vi "main.vi"() -> ()   [LabVIEW 2020]
uses:
  Typedefs/Queue_Operations.ctl
  Typedefs/Data Cluster.ctl
  Typedefs/Timer.ctl
  <vilib>/Utility/config.llb/Read Key (Double).vi
  <vilib>/Utility/config.llb/Write Key (Double).vi
  <vilib>/Utility/config.llb/NI_LVConfig.lvlib
panel:
  out "Milk Level":dbl(slide)=70.0 scale=0.0..100.0
  out "Bean Level":dbl(slide)=70.0 scale=0.0..100.0
  out "Water Level":dbl(slide)=70.0 scale=0.0..100.0
  in  "Power":bool
  out "Total Cups":dbl
  out "Elapsed Time":i32
  out "Dispensing":bool
  out "Brewing":bool
  out "Grinding":bool
  out "Heating":bool
  out "Purging":bool
  out "Dispenser":dbl(slide) scale=0.0..60.0
  out "Chamber":dbl(slide) scale=0.0..60.0
  out "Low Milk":bool
  out "Low Bean":bool
  out "Low Water":bool
  in  "Knob":i32(knob)=2 scale=0.0..2.0
  in  "1 Carafe":bool
  in  "1 Cup":bool
  out "Error out":errorcluster
  in  "Error in":errorcluster
  # "Coffee"
  # "Hot Water"
  # "Lattee"
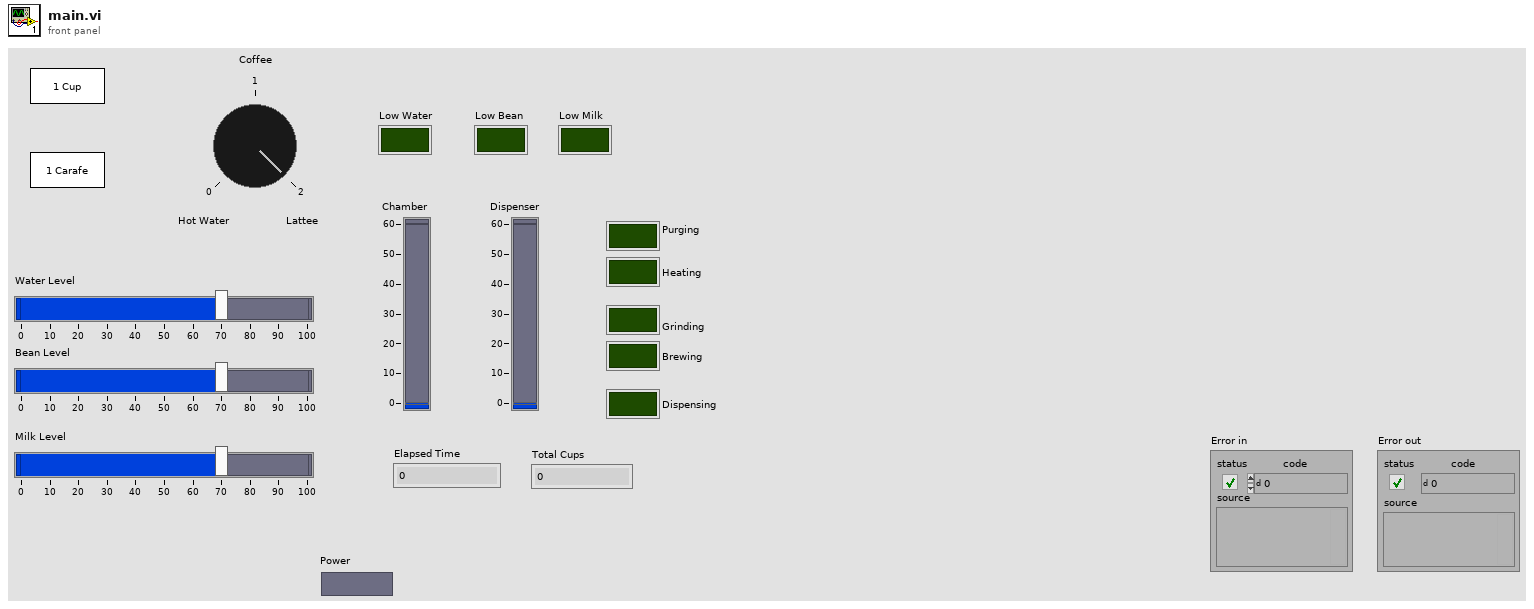
[diagram p1: front panel]
types:
  T1 = typedef "Data Cluster.ctl" = cluster{"Timer":T2, "Power":bool, "Total Cups":dbl, "Coffee Path":path, "Shut Down":dbl, "Water Level":dbl, "Bean Level":dbl, "Milk Level":dbl, "Knob":i32, "Beverage Type":string, "1 Cup":bool, "1 Carafe":bool, "Chamber":dbl, "Dispenser":dbl, "Set Time":dbl[], "Sequence":cluster{"Ingri":string, "Time":dbl}[], "index":i32, "Purging":bool, "Heating":bool, "Grinding":bool, "Brewing":bool, "Dispensing":bool, "Low Water":bool, "Low Bean":bool, "Low Milk":bool}
  T2 = typedef "Timer.ctl" = cluster{"Previous Time":dbl, "Elapsed Time":dbl, "Start":bool, "Pause?":bool}
  T3 = typedef "Queue_Operations.ctl" = enum16{"Obtain Queue", "Enqueue", "Enqueue N Element", "Enqueue at First", "Dequeue", "Release Queue", "Queue Status", "Flush Queue"}
  T4 = typedef "NI_LVConfig.lvlib/Config Data RefNum.ctl" = refnum<k1>
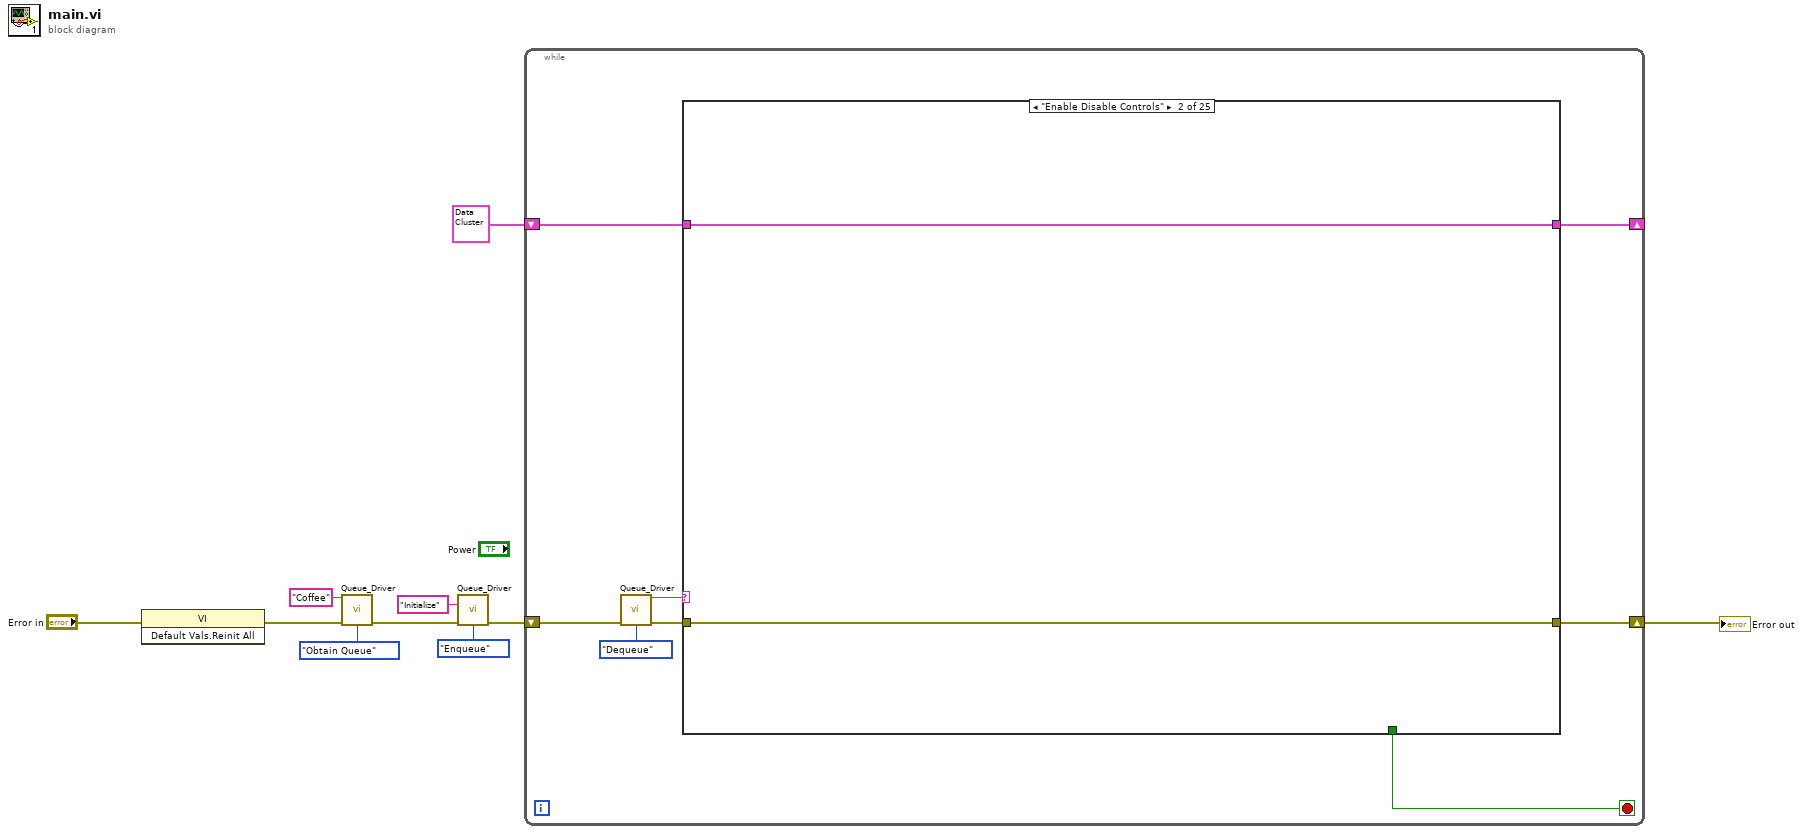
[diagram p0: block diagram]
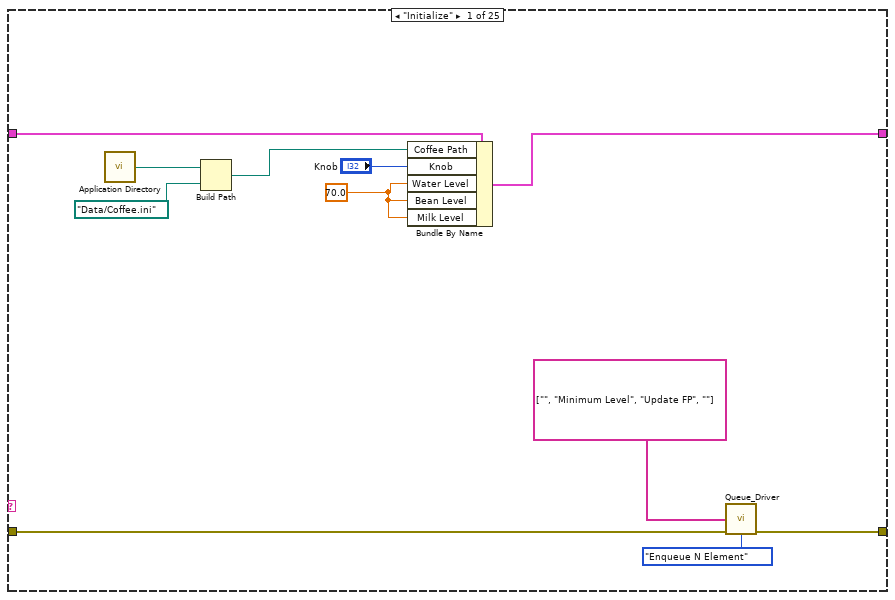
[diagram p2: hidden frame]
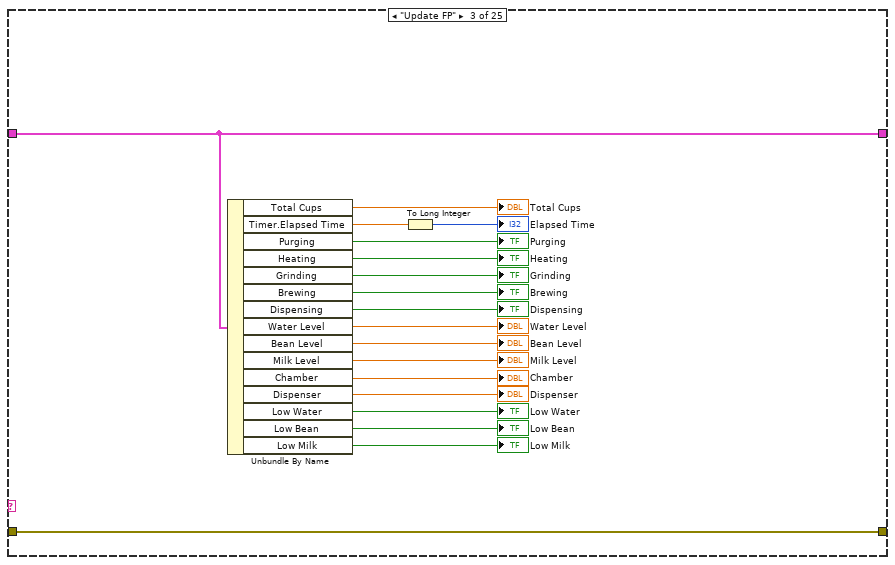
[diagram p3: hidden frame]
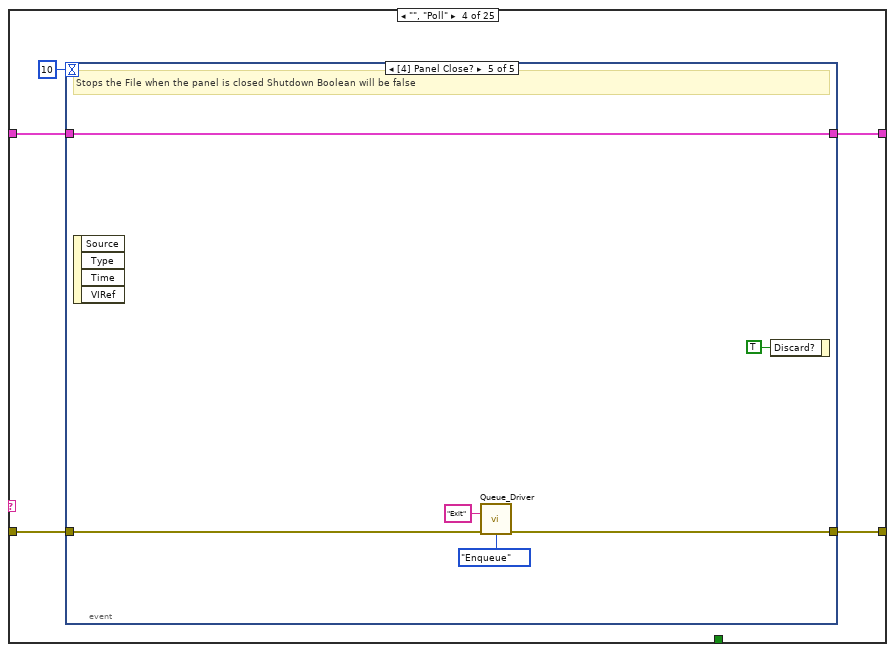
[diagram p4: hidden frame]
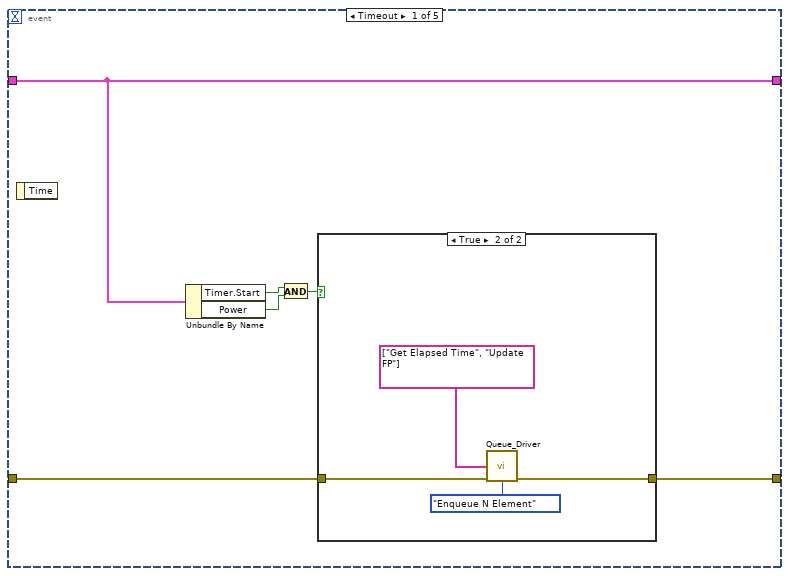
[diagram p5: hidden frame]
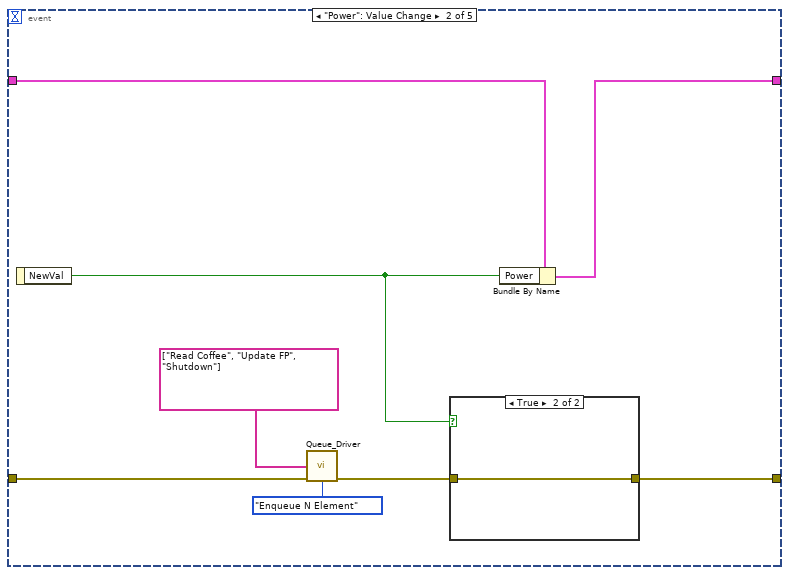
[diagram p7: hidden frame]
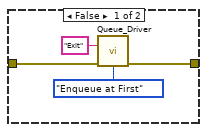
[diagram p8: hidden frame]
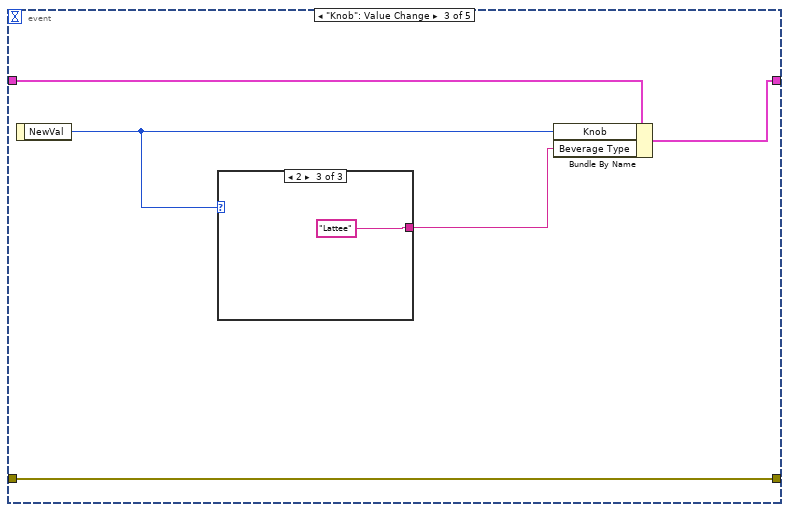
[diagram p9: hidden frame]
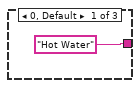
[diagram p10: hidden frame]
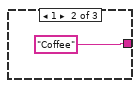
[diagram p11: hidden frame]
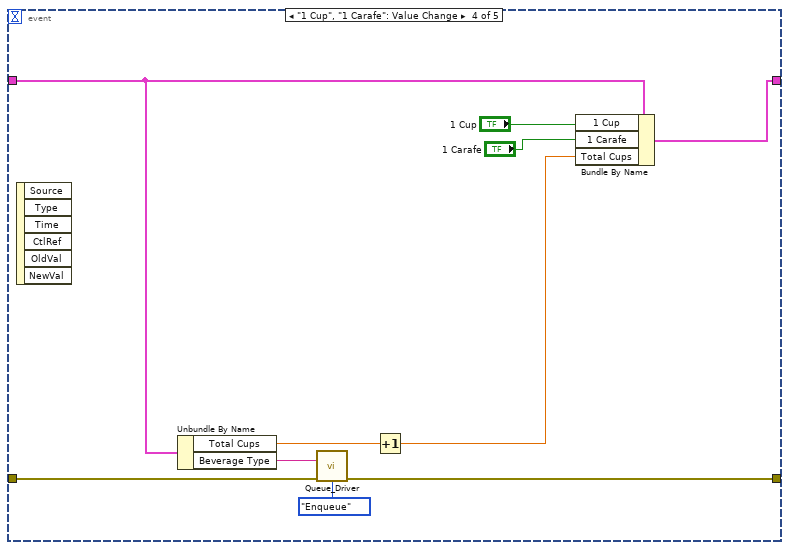
[diagram p12: hidden frame]
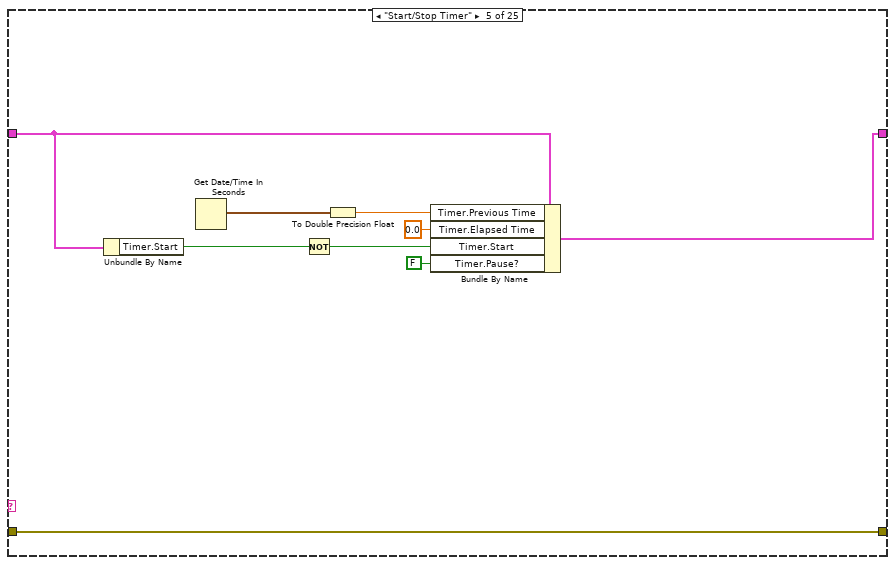
[diagram p13: hidden frame]
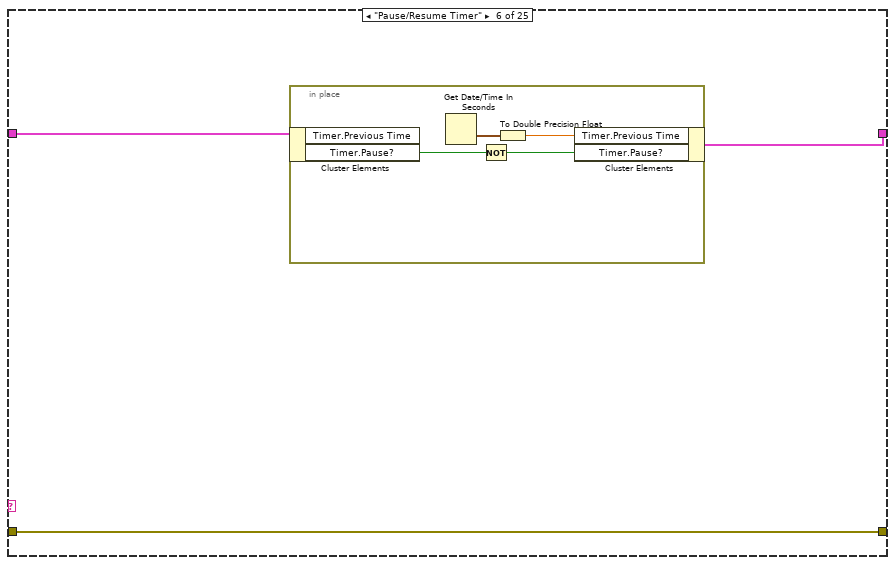
[diagram p14: hidden frame]
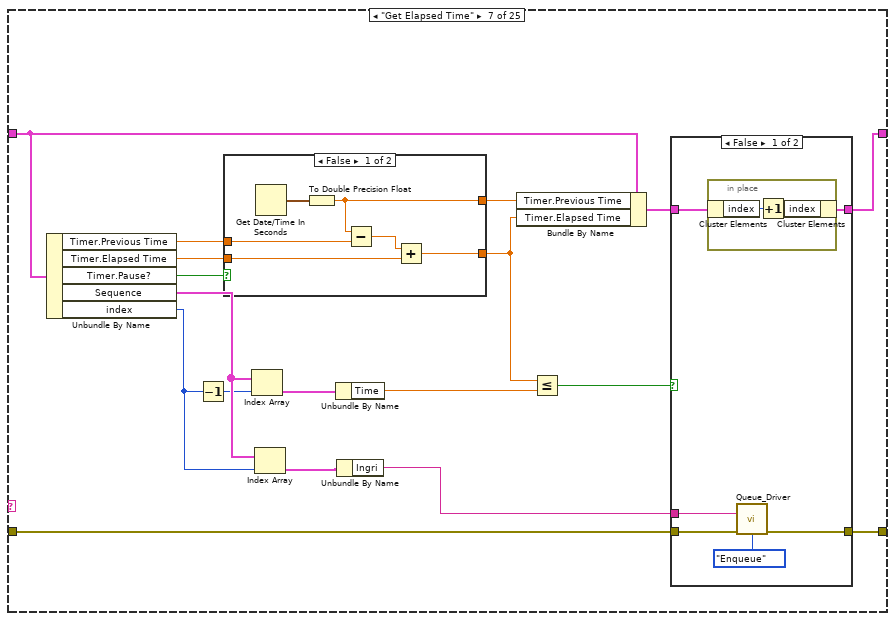
[diagram p15: hidden frame]
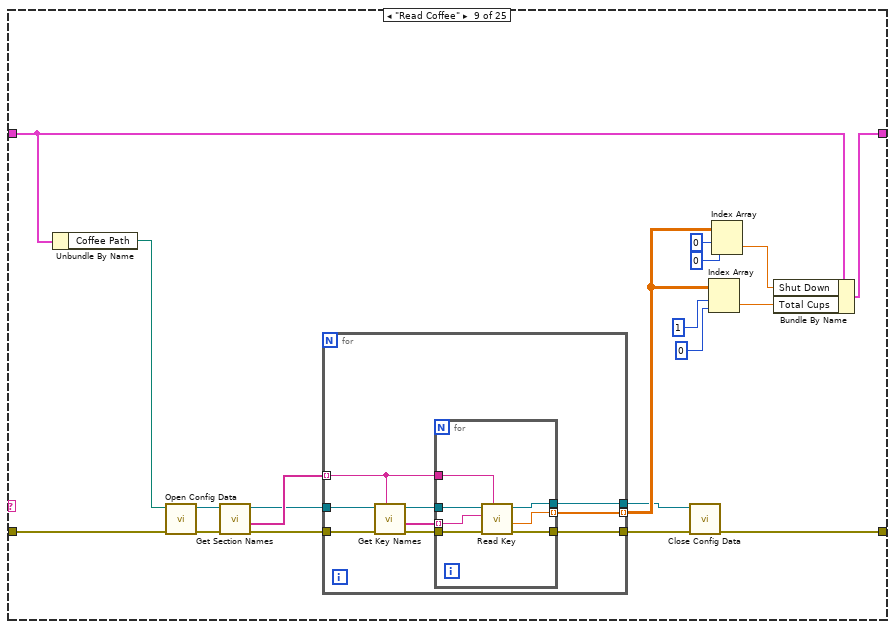
[diagram p19: hidden frame]
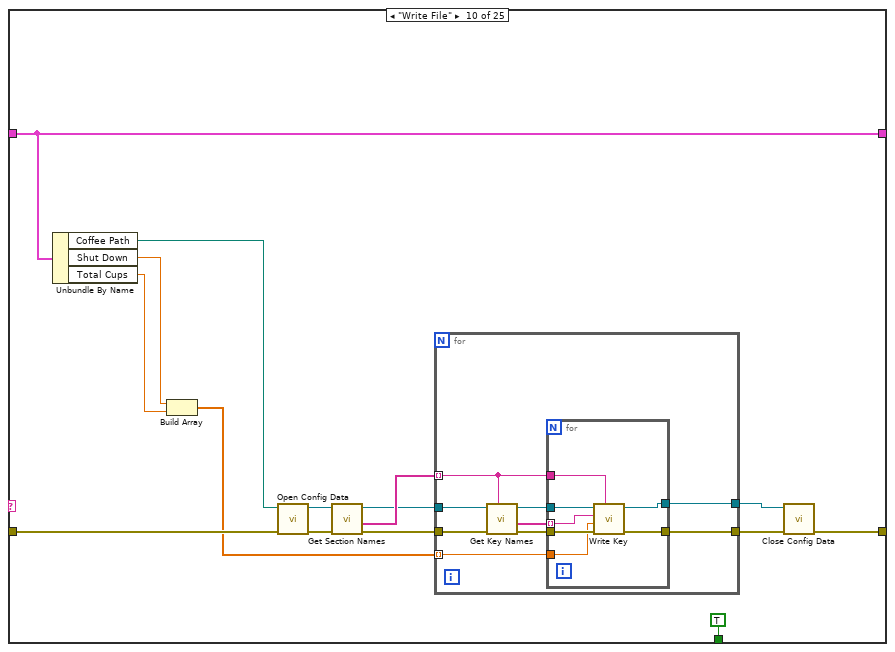
[diagram p20: hidden frame]
diagram:
  n1 = invoke class="VI" method="Default Vals.Reinit All"(error in="Error in") -> (error out=w1:errorcluster)  [unwired: 2 in, 2 out]
  n2 = call "Queue_Driver.vi"("Queue Name"="Coffee", "error in (no error)"=w1, "Queue Operation"=Queue_Operations."Obtain Queue") -> ("error out"=w6:errorcluster)  [unwired: 11 in, 1 out]
  n3 = call "Queue_Driver.vi"("Enqueue State"="Initialize", "error in (no error)"=w6, "Queue Operation"=Queue_Operations."Enqueue") -> ("error out"=w5:errorcluster)  [unwired: 11 in, 1 out]
  n4 = while {
    shift-right: [w18] -> w10
    shift-left: w5 -> [w17]
    shift-right: [w13] -> _
    shift-left: T1 {"Timer"={"Previous Time"=0.0, "Elapsed Time"=0.0, "Start"=FALSE, "Pause?"=FALSE}, "Power"=FALSE, "Total Cups"=0.0, "Coffee Path"=path "", "Shut Down"=0.0, "Water Level"=0.0, "Bean Level"=0.0, "Milk Level"=0.0, "Knob"=0, "Beverage Type"="", "1 Cup"=FALSE, "1 Carafe"=FALSE, "Chamber"=0.0, "Dispenser"=0.0, "Set Time"=[], "Sequence"=[{"Ingri"="Beverage Type", "Time"=0.0}], "index"=1, "Purging"=FALSE, "Heating"=FALSE, "Grinding"=FALSE, "Brewing"=FALSE, "Dispensing"=FALSE, "Low Water"=FALSE, "Low Bean"=FALSE, "Low Milk"=FALSE} ("Data Cluster") -> [w12]
    stop <- w11 stop-if-true
    n5 = call "Queue_Driver.vi"("error in (no error)"=w17, "Queue Operation"=Queue_Operations."Dequeue") -> ("Dequeued State"=w14:string, "error out"=w16:errorcluster)  [unwired: 12 in]
    n6 = case shown="\"Enable Disable Controls\"" w14 {
      tunnel: w16 -> [w23 w30 w49 w54 w103 w112 w130 w155 w172 w205 w229 w250 w255 w263 w272 w281 w306 w327 w358 w365 w374 w380 w390 w396 w398]
      tunnel: [w24 w30 w49 w53 w103 w112 w131 w155 w158 w194 w223 w250 w254 w262 w271 w281 w306 w327 w358 w365 w374 w379 w389 w396 w398] -> w18
      tunnel: [w28 w31 w48 w51 w111 w113 w120 w156 w175 w199 w232 w244 w257 w265 w274 w280 w308 w330 w359 w363 w373 w384 w393 w397 w399] -> w13
      tunnel: w12 -> [w29 w31 w48 w52 w106 w114 w133 w156 w174 w199 w234 w245 w258 w266 w268 w276 w303 w324 w354 w364 w367 w382 w395 w397 w399]
      tunnel: [_ _ _ _ _ _ _ _ _ TRUE _ _ _ _ _ _ _ _ _ _ _ _ FALSE _ _] -> w11
      frame "Initialize" {
        w19 = 70.0 ("Water Level")
        n7 = call <vilib>:"Application Directory.vi"() -> ("Application Directory"=w27:path)
        n8 = Build Path(base path=w27, name or relative path=path "Data/Coffee.ini") -> (appended path=w25:path)
        n9 = Bundle By Name(cluster=w29, "Coffee Path"=w25, "Knob"="Knob", "Water Level"=w19, "Bean Level"=w19, "Milk Level"=w19) -> (w28:T1)
        n10 = call "Queue_Driver.vi"("Array of States"=string[] ["", "Minimum Level", "Update FP", ""], "error in (no error)"=w23, "Queue Operation"=Queue_Operations."Enqueue N Element") -> ("error out"=w24:errorcluster)  [unwired: 11 in, 1 out]
      }
      frame "Enable Disable Controls" {
      }
      frame "Update FP" {
        n11 = Unbundle By Name(w48) -> ("Total Cups"=→"Total Cups":dbl, "Timer.Elapsed Time"=w47:dbl, "Purging"=→"Purging":bool, "Heating"=→"Heating":bool, "Grinding"=→"Grinding":bool, "Brewing"=→"Brewing":bool, "Dispensing"=→"Dispensing":bool, "Water Level"=→"Water Level":dbl, "Bean Level"=→"Bean Level":dbl, "Milk Level"=→"Milk Level":dbl, "Chamber"=→"Chamber":dbl, "Dispenser"=→"Dispenser":dbl, "Low Water"=→"Low Water":bool, "Low Bean"=→"Low Bean":bool, "Low Milk"=→"Low Milk":bool)
        n12 = To Long Integer(number=w47) -> (32bit integer=→"Elapsed Time":i32)
      }
      frame "", "Poll" {
        n13 = event shown="[4] Panel Close?" {
          selector: _ -> [_ _ _ _ _]
          dyn-events: _ -> [_ _ _ _ _]
          timeout: 10 -> [_ _ _ _ _]
          tunnel: w54 -> [w60 w71 w81 w96 w100]
          tunnel: [w59 w67 w81 w95 w99] -> w53
          tunnel: w52 -> [w58 w73 w83 w92 w102]
          tunnel: [w58 w72 w82 w91 w102] -> w51
          event Timeout {
            n14 = event-data() -> ()  [unwired: 1 in, 1 out]
            n15 = Unbundle By Name(w58) -> ("Timer.Start"=w56:bool, "Power"=w55:bool)
            n16 = And(x=w56, y=w55) -> (x .and. y?=w57:bool)
            n17 = case shown="True" w57 {
              tunnel: w60 -> [w61 w65]
              tunnel: [w61 w64] -> w59
              frame False {
              }
              frame True {
                n18 = call "Queue_Driver.vi"("Array of States"=string[] ["Get Elapsed Time", "Update FP"], "error in (no error)"=w65, "Queue Operation"=Queue_Operations."Enqueue N Element") -> ("error out"=w64:errorcluster)  [unwired: 11 in, 1 out]
              }
            }
          }
          event "Power": Value Change {
            n19 = event-data() -> ("NewVal"=w66:bool)  [unwired: 1 in]
            n20 = call "Queue_Driver.vi"("Array of States"=string[] ["Read Coffee", "Update FP", "Shutdown"], "error in (no error)"=w71, "Queue Operation"=Queue_Operations."Enqueue N Element") -> ("error out"=w68:errorcluster)  [unwired: 11 in, 1 out]
            n21 = case shown="True" w66 {
              tunnel: w68 -> [w77 w78]
              tunnel: [w76 w78] -> w67
              frame False {
                n22 = call "Queue_Driver.vi"("Enqueue State"="Exit", "error in (no error)"=w77, "Queue Operation"=Queue_Operations."Enqueue at First") -> ("error out"=w76:errorcluster)  [unwired: 11 in, 1 out]
              }
              frame True {
              }
            }
            n23 = Bundle By Name(cluster=w73, "Power"=w66) -> (w72:T1)
          }
          event "Knob": Value Change {
            n24 = event-data() -> ("NewVal"=w80:i32)  [unwired: 1 in]
            n25 = case shown="2" w80 {
              tunnel: ["Hot Water" "Coffee" "Lattee"] -> w79
              frame 0, Default {
              }
              frame 1 {
              }
              frame 2 {
              }
            }
            n26 = Bundle By Name(cluster=w83, "Knob"=w80, "Beverage Type"=w79) -> (w82:T1)
          }
          event "1 Cup", "1 Carafe": Value Change {
            n27 = event-data() -> ()  [unwired: 1 in, 6 out]
            n28 = Unbundle By Name(w92) -> ("Total Cups"=w88:dbl, "Beverage Type"=w93:string)
            n29 = call "Queue_Driver.vi"("Enqueue State"=w93, "error in (no error)"=w96, "Queue Operation"=Queue_Operations."Enqueue") -> ("error out"=w95:errorcluster)  [unwired: 11 in, 1 out]
            n30 = Increment(x=w88) -> (x+1=w87:dbl)
            n31 = Bundle By Name(cluster=w92, "1 Cup"="1 Cup", "1 Carafe"="1 Carafe", "Total Cups"=w87) -> (w91:T1)
          }
          event Panel Close? {
            # "Stops the File when the panel is closed Shutdown Boolean will be false"
            n32 = event-data() -> ()  [unwired: 1 in, 4 out]
            n33 = call "Queue_Driver.vi"("Enqueue State"="Exit", "error in (no error)"=w100, "Queue Operation"=Queue_Operations."Enqueue") -> ("error out"=w99:errorcluster)  [unwired: 11 in, 1 out]
            n34 = event-data("Discard?"=TRUE) -> ()  [unwired: 1 in, 1 out]
          }
        }
      }
      frame "Start/Stop Timer" {
        n35 = Unbundle By Name(w106) -> ("Timer.Start"=w105:bool)
        n36 = Get Date/Time In Seconds() -> (seconds since 1Jan1904=w109:timestamp)
        n37 = Not(x=w105) -> (.not. x?=w104:bool)
        n38 = To Double Precision Float(number=w109) -> (double precision float=w110:dbl)
        n39 = Bundle By Name(cluster=w106, "Timer.Previous Time"=w110, "Timer.Elapsed Time"=0.0, "Timer.Start"=w104, "Timer.Pause?"=FALSE) -> (w111:T1)
      }
      frame "Pause/Resume Timer" {
        n40 = in-place {
          n41 = in-place-cluster #1(w114) -> ("Timer.Pause?"=w116:bool)  [unwired: 1 out]
          n42 = Get Date/Time In Seconds() -> (seconds since 1Jan1904=w118:timestamp)
          n43 = Not(x=w116) -> (.not. x?=w115:bool)
          n44 = To Double Precision Float(number=w118) -> (double precision float=w117:dbl)
          n45 = in-place-cluster #1("Timer.Previous Time"=w117, "Timer.Pause?"=w115) -> (w113:T1)
        }
      }
      frame "Get Elapsed Time" {
        n46 = Unbundle By Name(w133) -> ("Timer.Previous Time"=w136:dbl, "Timer.Elapsed Time"=w135:dbl, "Timer.Pause?"=w134:bool, "Sequence"=w125:cluster{"Ingri":string, "Time":dbl}[], "index"=w124:i32)
        n47 = Decrement(x=w124) -> (x-1=w119:i32)
        n48 = case shown="False" w134 {
          tunnel: w136 -> [w152 w154]
          tunnel: w135 -> [w149 w153]
          tunnel: [w148 w153] -> w128
          tunnel: [w147 w154] -> w132
          frame False {
            n49 = Get Date/Time In Seconds() -> (seconds since 1Jan1904=w151:timestamp)
            n50 = To Double Precision Float(number=w151) -> (double precision float=w147:dbl)
            n51 = Subtract(x=w147, y=w152) -> (x-y=w150:dbl)
            n52 = Add(x=w150, y=w149) -> (x+y=w148:dbl)
          }
          frame True {
          }
        }
        n53 = Index Array(array=w125, index=w119) -> (element=w129:cluster{"Ingri":string, "Time":dbl})
        n54 = Index Array(array=w125, index=w124) -> (element=w123:cluster{"Ingri":string, "Time":dbl})
        n55 = Unbundle By Name(w129) -> ("Time"=w127:dbl)
        n56 = Unbundle By Name(w123) -> ("Ingri"=w122:string)
        n57 = Bundle By Name(cluster=w133, "Timer.Previous Time"=w132, "Timer.Elapsed Time"=w128) -> (w121:T1)
        n58 = Less Or Equal?(x=w128, y=w127) -> (x <= y?=w126:bool)
        n59 = case shown="False" w126 {
          tunnel: [w139 w146] -> w131
          tunnel: w130 -> [w142 w146]
          tunnel: w122 -> [w140 _]
          tunnel: w121 -> [w138 w145]
          tunnel: [w137 w145] -> w120
          frame False {
            n60 = in-place {
              n61 = in-place-cluster #2(w138) -> ("index"=w144:i32)
              n62 = Increment(x=w144) -> (x+1=w143:i32)
              n63 = in-place-cluster #2("index"=w143) -> (w137:T1)
            }
            n64 = call "Queue_Driver.vi"("Enqueue State"=w140, "error in (no error)"=w142, "Queue Operation"=Queue_Operations."Enqueue") -> ("error out"=w139:errorcluster)  [unwired: 11 in, 1 out]
          }
          frame True {
          }
        }
      }
      frame "Read File" {
      }
      frame "Read Coffee" {
        n65 = Unbundle By Name(w174) -> ("Coffee Path"=w173:path)
        n66 = call <vilib>:"Open Config Data.vi"("error in (no error)"=w172, "configuration file path"=w173) -> ("error out"=w171:errorcluster, "refnum"=w170:T4)  [unwired: 7 in, 1 out]
        n67 = call <vilib>:"Get Section Names.vi"("error in (no error)"=w171, "refnum"=w170) -> ("error out"=w168:errorcluster, "section names"=w169:string[], "refnum out"=w167:T4)  [unwired: 7 in]
        n68 = for {
          tunnel: w169 -> [w177] mode=indexing
          tunnel: [w183] -> w163 mode=indexing
          tunnel: w168 -> [w182]
          tunnel: [w180] -> w159
          tunnel: w167 -> [w179]
          tunnel: [w176] -> w157
          n69 = call <vilib>:"Get Key Names.vi"("section"=w177, "error in (no error)"=w182, "refnum"=w179) -> ("error out"=w181:errorcluster, "key names"=w184:string[], "refnum out"=w178:T4)  [unwired: 5 in, 1 out]
          n70 = for {
            tunnel: w184 -> [w191] mode=indexing
            tunnel: [w190] -> w183 mode=indexing
            tunnel: w181 -> [w189]
            tunnel: [w188] -> w180
            tunnel: w178 -> [w187]
            tunnel: w177 -> [w186]
            tunnel: [w185] -> w176
            n71 = call-poly <vilib>:"Read Key.vi"("section"=w186, "error in (no error)"=w189, "key"=w191, "refnum"=w187) -> ("error out"=w188:errorcluster, "value"=w190:dbl, "refnum out"=w185:T4)  [unwired: 4 in, 1 out]
          }
        }
        n72 = call <vilib>:"Close Config Data.vi"("error in (no error)"=w159, "refnum"=w157) -> ("error out"=w158:errorcluster)  [unwired: 8 in, 1 out]
        n73 = Index Array(array=w163, index (row)=1, index (col)=0 ("disabled index (col)")) -> (element=w164:dbl)
        n74 = Index Array(array=w163, index (row)=0, index (col)=0 ("disabled index (col)")) -> (element=w160:dbl)
        n75 = Bundle By Name(cluster=w174, "Shut Down"=w160, "Total Cups"=w164) -> (w175:T1)
      }
      frame "Write File" {
        n76 = Unbundle By Name(w199) -> ("Coffee Path"=w206:path, "Shut Down"=w198:dbl, "Total Cups"=w197:dbl)
        n77 = Build Array(w198, w197) -> (w196:dbl[])
        n78 = call <vilib>:"Open Config Data.vi"("error in (no error)"=w205, "configuration file path"=w206) -> ("error out"=w204:errorcluster, "refnum"=w203:T4)  [unwired: 7 in, 1 out]
        n79 = call <vilib>:"Get Section Names.vi"("error in (no error)"=w204, "refnum"=w203) -> ("error out"=w201:errorcluster, "section names"=w202:string[], "refnum out"=w200:T4)  [unwired: 7 in]
        n80 = for {
          tunnel: w202 -> [w209] mode=indexing
          tunnel: w201 -> [w214]
          tunnel: [w212] -> w195
          tunnel: w200 -> [w211]
          tunnel: w196 -> [w207] mode=indexing
          tunnel: [w208] -> w193
          n81 = call <vilib>:"Get Key Names.vi"("section"=w209, "error in (no error)"=w214, "refnum"=w211) -> ("error out"=w213:errorcluster, "key names"=w215:string[], "refnum out"=w210:T4)  [unwired: 5 in, 1 out]
          n82 = for {
            tunnel: w215 -> [w222] mode=indexing
            tunnel: w213 -> [w221]
            tunnel: [w220] -> w212
            tunnel: w210 -> [w219]
            tunnel: w209 -> [w218]
            tunnel: [w217] -> w208
            tunnel: w207 -> [w216]
            n83 = call-poly <vilib>:"Write Key.vi"("section"=w218, "error in (no error)"=w221, "value"=w216, "key"=w222, "refnum"=w219) -> ("error out"=w220:errorcluster, "refnum out"=w217:T4)  [unwired: 4 in, 1 out]
          }
        }
        n84 = call <vilib>:"Close Config Data.vi"("error in (no error)"=w195, "refnum"=w193) -> ("error out"=w194:errorcluster)  [unwired: 8 in, 1 out]
      }
      frame "Shutdown" {
        n85 = Unbundle By Name(w234) -> ("Shut Down"=w233:dbl)
        n86 = Equal To 0?(x=w233) -> (x = 0?=w230:bool)
        n87 = case shown="True" w230 {
          tunnel: [cluster{"Ingri":string, "Time":dbl}[] [{"Ingri"="Purging", "Time"=4.0}, {"Ingri"="Heating", "Time"=5.0}] ("Sequence") cluster{"Ingri":string, "Time":dbl}[] [{"Ingri"="Heating", "Time"=5.0}, {"Ingri"="", "Time"=0.0}] ("Sequence")] -> w231
          tunnel: ["Purging" ("Beverage Type") "Heating" ("Beverage Type")] -> w224
          frame True {
          }
          frame False {
          }
        }
        n88 = call "Queue_Driver.vi"("Enqueue State"="Start/Stop Timer", "error in (no error)"=w229, "Queue Operation"=Queue_Operations."Enqueue") -> ("error out"=w226:errorcluster)  [unwired: 11 in, 1 out]
        n89 = call "Queue_Driver.vi"("Enqueue State"=w224, "error in (no error)"=w226, "Queue Operation"=Queue_Operations."Enqueue") -> ("error out"=w223:errorcluster)  [unwired: 11 in, 1 out]
        n90 = Bundle By Name(cluster=w234, "Sequence"=w231) -> (w232:T1)
      }
      frame "Minimum Level" {
        w246 = 30.0 ("y")
        n91 = Unbundle By Name(w245) -> ("Water Level"=w249:dbl, "Bean Level"=w248:dbl, "Milk Level"=w247:dbl)
        n92 = Less Or Equal?(x=w249, y=w246) -> (x <= y?=w243:bool)
        n93 = Less Or Equal?(x=w248, y=w246) -> (x <= y?=w242:bool)
        n94 = Less Or Equal?(x=w247, y=w246) -> (x <= y?=w241:bool)
        n95 = Build Array(w243, w242, w241) -> (w240:bool[])
        n96 = Boolean Array To Number(Boolean array=w240) -> (number=w239:u32)
        n97 = case shown="7" w239 {
          frame 0, 1, 4, 6 {
          }
          frame 7 {
          }
          frame 3 {
          }
          frame 5 {
          }
          frame 1000, Default {
          }
        }
        n98 = Bundle By Name(cluster=w245, "Low Water"=w243, "Low Bean"=w242, "Low Milk"=w241) -> (w244:T1)
      }
      frame "Coffee" {
        n99 = Bundle By Name(cluster=w258, "Sequence"=cluster{string, dbl}[] [{"Bean", 3.0}, {"Water", 4.0}, {"Dispensing", 5.0}] ("Array 2"), "Timer.Elapsed Time"=0.0) -> (w257:T1)
        n100 = call "Queue_Driver.vi"("Array of States"=string[] ["Start/Stop Timer", "Bean"], "error in (no error)"=w255, "Queue Operation"=Queue_Operations."Enqueue N Element") -> ("error out"=w254:errorcluster)  [unwired: 11 in, 1 out]
      }
      frame "Lattee" {
        n101 = call "Queue_Driver.vi"("Array of States"=string[] ["Start/Stop Timer", "Bean"], "error in (no error)"=w263, "Queue Operation"=Queue_Operations."Enqueue N Element") -> ("error out"=w262:errorcluster)  [unwired: 11 in, 1 out]
        n102 = Bundle By Name(cluster=w266, "Sequence"=cluster{string, dbl}[] [{"Bean", 3.0}, {"Milk", 0.0}, {"Water", 4.0}, {"Dispensing", 5.0}] ("Array 2"), "Timer.Elapsed Time"=0.0) -> (w265:T1)
      }
      frame "Hot Water" {
        n103 = call "Queue_Driver.vi"("Array of States"=string[] ["Start/Stop Timer", "Dispensing"], "error in (no error)"=w272, "Queue Operation"=Queue_Operations."Enqueue N Element") -> ("error out"=w271:errorcluster)  [unwired: 11 in, 1 out]
        n104 = Bundle By Name(cluster=w268, "Sequence"=cluster{string, dbl}[] [{"Dispensing", 5.0}, {"", 0.0}, {"", 0.0}] ("Array 2"), "Timer.Elapsed Time"=0.0) -> (w274:T1)
      }
      frame "Bean" {
        w278 = FALSE ("Purging")
        n105 = Unbundle By Name(w276) -> ("1 Cup"=w277:bool)
        n106 = case shown="True" w277 {
          tunnel: w276 -> [w283 w290]
          tunnel: [w282 w289] -> w275
          frame True {
            n107 = in-place {
              w286 = 5.0 ("y")
              n108 = in-place-cluster #3(w283) -> ("Chamber"=w285:dbl, "Bean Level"=w288:dbl)
              n109 = Subtract(x=w288, y=w286) -> (x-y=w287:dbl)
              n110 = Add(x=w285, y=w286) -> (x+y=w284:dbl)
              n111 = in-place-cluster #3("Chamber"=w284, "Bean Level"=w287) -> (w282:T1)
            }
          }
          frame False {
            n112 = in-place {
              w293 = 20.0 ("y")
              n113 = in-place-cluster #4(w290) -> ("Chamber"=w292:dbl, "Bean Level"=w295:dbl)
              n114 = Subtract(x=w295, y=w293) -> (x-y=w294:dbl)
              n115 = Add(x=w292, y=w293) -> (x+y=w291:dbl)
              n116 = in-place-cluster #4("Chamber"=w291, "Bean Level"=w294) -> (w289:T1)
            }
          }
        }
        n117 = Bundle By Name(cluster=w275, "Purging"=w278, "Heating"=w278, "Grinding"=TRUE, "Brewing"=w278, "Dispensing"=w278) -> (w280:T1)
      }
      frame "Water" {
        w307 = FALSE ("Purging")
        n118 = Unbundle By Name(w303) -> ("1 Cup"=w302:bool, "Knob"=w301:i32)
        n119 = case shown="True" w302 {
          tunnel: w303 -> [w310 w317]
          tunnel: [w309 w316] -> w304
          frame True {
            n120 = in-place {
              w313 = 5.0 ("y")
              n121 = in-place-cluster #5(w310) -> ("Chamber"=w312:dbl, "Water Level"=w315:dbl)
              n122 = Subtract(x=w315, y=w313) -> (x-y=w314:dbl)
              n123 = Add(x=w312, y=w313) -> (x+y=w311:dbl)
              n124 = in-place-cluster #5("Chamber"=w311, "Water Level"=w314) -> (w309:T1)
            }
          }
          frame False {
            n125 = in-place {
              w320 = 20.0 ("y")
              n126 = in-place-cluster #6(w317) -> ("Chamber"=w319:dbl, "Water Level"=w322:dbl)
              n127 = Subtract(x=w322, y=w320) -> (x-y=w321:dbl)
              n128 = Add(x=w319, y=w320) -> (x+y=w318:dbl)
              n129 = in-place-cluster #6("Chamber"=w318, "Water Level"=w321) -> (w316:T1)
            }
          }
        }
        n130 = Equal To 0?(x=w301) -> (x = 0?=w299:bool)
        n131 = Select(t=5.0, s=w299, f=0.0) -> (s? t:f=w296:dbl)
        n132 = Not(x=w299) -> (.not. x?=w300:bool)
        n133 = Bundle By Name(cluster=w304, "Purging"=w307, "Heating"=w307, "Grinding"=w307, "Brewing"=w300, "Dispensing"=w299, "Timer.Elapsed Time"=0.0, "Dispenser"=w296) -> (w308:T1)
      }
      frame "Milk" {
        w328 = FALSE ("Purging")
        n134 = Unbundle By Name(w324) -> ("1 Cup"=w323:bool)
        n135 = case shown="True" w323 {
          tunnel: w324 -> [w332 w339]
          tunnel: [w331 w338] -> w325
          frame True {
            n136 = in-place {
              w335 = 5.0 ("y")
              n137 = in-place-cluster #7(w332) -> ("Chamber"=w334:dbl, "Milk Level"=w337:dbl)
              n138 = Subtract(x=w337, y=w335) -> (x-y=w336:dbl)
              n139 = Add(x=w334, y=w335) -> (x+y=w333:dbl)
              n140 = in-place-cluster #7("Chamber"=w333, "Milk Level"=w336) -> (w331:T1)
            }
          }
          frame False {
            n141 = in-place {
              w342 = 20.0 ("y")
              n142 = in-place-cluster #8(w339) -> ("Chamber"=w341:dbl, "Milk Level"=w344:dbl)
              n143 = Subtract(x=w344, y=w342) -> (x-y=w343:dbl)
              n144 = Add(x=w341, y=w342) -> (x+y=w340:dbl)
              n145 = in-place-cluster #8("Chamber"=w340, "Milk Level"=w343) -> (w338:T1)
            }
          }
        }
        n146 = Bundle By Name(cluster=w325, "Purging"=w328, "Heating"=w328, "Grinding"=w328, "Brewing"=TRUE, "Dispensing"=w328, "Timer.Elapsed Time"=0.0) -> (w330:T1)
      }
      frame "Dispensing" {
        w356 = FALSE ("Purging")
        n147 = Unbundle By Name(w354) -> ("Knob"=w347:i32, "Chamber"=w349:dbl, "Sequence"=w353:cluster{"Ingri":string, "Time":dbl}[])
        n148 = Insert Into Array(array=w353, new element=cluster{"Ingri":string, "Time":dbl} {"Ingri"="End", "Time"=3.0} ("new element/subarray")) -> (w351:cluster{"Ingri":string, "Time":dbl}[])  [unwired: 1 in]
        n149 = Equal To 0?(x=w347) -> (x = 0?=w348:bool)
        n150 = Select(t=5.0, s=w348, f=w349) -> (s? t:f=w345:dbl)
        n151 = Bundle By Name(cluster=w354, "Chamber"=0.0, "Dispenser"=w345, "Purging"=w356, "Heating"=w356, "Grinding"=w356, "Brewing"=w356, "Dispensing"=TRUE, "Timer.Elapsed Time"=0.0, "Sequence"=w351) -> (w359:T1)
      }
      frame "Purging" {
        w361 = FALSE ("Heating")
        n152 = Bundle By Name(cluster=w364, "Purging"=TRUE, "Heating"=w361, "Grinding"=w361, "Brewing"=w361, "Dispensing"=w361, "Timer.Elapsed Time"=0.0) -> (w363:T1)
      }
      frame "Heating" {
        w372 = FALSE ("Heating")
        n153 = Unbundle By Name(w367) -> ("Sequence"=w366:cluster{"Ingri":string, "Time":dbl}[])
        n154 = Insert Into Array(array=w366, new element=cluster{"Ingri":string, "Time":dbl} {"Ingri"="End", "Time"=3.0} ("new element/subarray")) -> (w368:cluster{"Ingri":string, "Time":dbl}[])  [unwired: 1 in]
        n155 = Bundle By Name(cluster=w367, "Purging"=w372, "Heating"=TRUE, "Grinding"=w372, "Brewing"=w372, "Dispensing"=w372, "Timer.Elapsed Time"=0.0, "Sequence"=w368) -> (w373:T1)
      }
      frame "End" {
        w381 = FALSE ("Purging")
        n156 = call "Queue_Driver.vi"("Array of States"=string[] ["Start/Stop Timer", "Update FP"], "error in (no error)"=w380, "Queue Operation"=Queue_Operations."Enqueue N Element") -> ("error out"=w379:errorcluster)  [unwired: 11 in, 1 out]
        n157 = Bundle By Name(cluster=w382, "Purging"=w381, "Heating"=w381, "Grinding"=w381, "Brewing"=w381, "Dispensing"=w381, "Timer.Elapsed Time"=0.0, "Dispenser"=0.0, "index"=1) -> (w384:T1)
      }
      frame "Exit" {
        n158 = Unbundle By Name(w395) -> ("Power"=w394:bool)
        n159 = Not(x=w394) -> (.not. x?=w385:bool)
        n160 = Boolean To (0,1)(Boolean=w385) -> (0, 1=w392:i16)
        n161 = To Double Precision Float(number=w392) -> (double precision float=w391:dbl)
        n162 = call "Queue_Driver.vi"("Enqueue State"="Write File", "error in (no error)"=w390, "Queue Operation"=Queue_Operations."Enqueue") -> ("error out"=w389:errorcluster)  [unwired: 11 in, 1 out]
        n163 = Bundle By Name(cluster=w395, "Shut Down"=w391) -> (w393:T1)
      }
      frame "Error" {
      }
      frame "Developer Case", Default {
      }
    }
  }
  "Error out" <- w10
